vi "全局 1.vi"() -> ()   [LabVIEW 2017]
panel:
  in  "XYGraph引用句柄":refnum<vi>
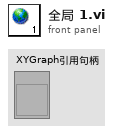
[diagram p1: front panel]
diagram:
